vi "SVL AC & DC Level (1 Ch DBL WDT).vi"(9 "window":u16(ring)=8 items=["None ", "Hanning", "Hamming", "Blackman-Harris", "Exact Blackman", "Blackman", "Flat Top", "4 Term B-Harris ", "7 Term B-Harris", "Low Sidelobe"], 11 "scaled signal [EU]":waveform(dbl)={"t0"=timestamp(0 s since 1904-01-01), "dt"=0.0, "Y"=[]}) -> (1 "DC level [EU]":dbl=nan format="%0.2f", 2 "AC level [EU rms]":dbl=nan format="%.8f", 3 "AC signal [EU]":waveform(dbl))   [LabVIEW 2017]
doc: "Computes the AC level and DC level of a signal. Wire data to the <B>scaled signal [EU]</B> input to determine the polymorphic instance to use or manually select the instance."
uses:
  <vilib>/Analysis/baseanly.llb/Mean (DBL).vi
  <vilib>/Analysis/0measdsp.llb/Scaled Time Domain Window (DBL).vi
  <vilib>/Analysis/NI_AALBase.lvlib
  <vilib>/Analysis/NI_AALPro.lvlib
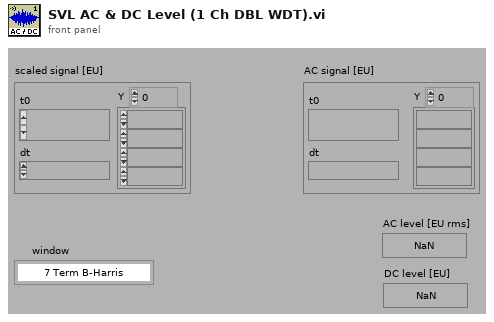
[diagram p1: front panel]
types:
  T1 = typedef "NI_AALPro.lvlib/windowTd.ctl" = u32
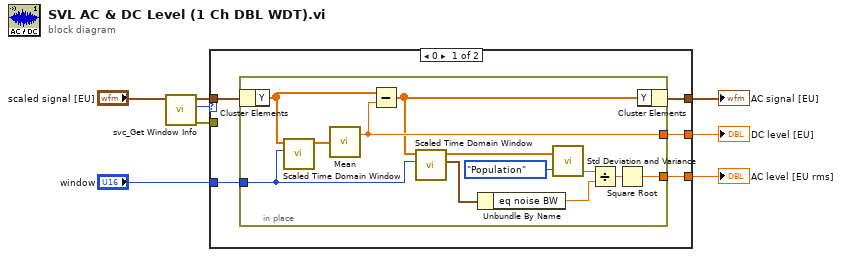
[diagram p0: block diagram]
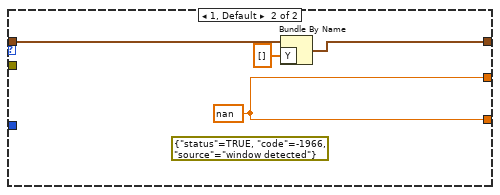
[diagram p2: hidden frame]
diagram:
  n1 = call <vilib>:"svc_Get Window Info.vi"("scaled signal [EU]"="scaled signal [EU]") -> ("error out"=w2:errorcluster, "window"=w1:T1, "dup scaled signal [EU]"=w3:waveform(dbl))  [unwired: 6 in, 2 out]
  n2 = case shown="0" w1 {
    tunnel: [w12 w29] -> w8
    tunnel: [w11 w29] -> w4
    tunnel: "window" -> [w13 _]
    tunnel: [w10 w27] -> w6
    tunnel: w3 -> [w9 w28]
    tunnel: w2 -> [_ _]
    frame 0 {
      n3 = in-place {
        in-place-border: [w19] -> w11
        in-place-border: w13 -> [w14]
        in-place-border: [w20] -> w12
        n4 = in-place-cluster #1(w9) -> ("Y"=w25:dbl[])
        n5 = call-poly <vilib>:"Scaled Time Domain Window.vi"("window"=w14, "X"=w25) -> ("Windowed X"=w18:dbl[])  [unwired: 7 in, 2 out]
        n6 = call-poly <vilib>:"Mean.vi"("X"=w18) -> ("mean"=w19:dbl)  [unwired: 1 out]
        n7 = Subtract(x=w25, y=w19) -> (x-y=w16:dbl[])
        n8 = call-poly <vilib>:"Scaled Time Domain Window.vi"("window"=w14, "X"=w16) -> ("window properties"=w15:cluster{"eq noise BW":dbl, "coherent gain":dbl}, "Windowed X"=w17:dbl[])  [unwired: 7 in, 1 out]
        n9 = Unbundle By Name(w15) -> ("eq noise BW"=w21:dbl)
        n10 = call <vilib>:"Std Deviation and Variance.vi"("X"=w17, "Weighting (Sample)"=enum16{"Sample", "Population"}."Population") -> ("variance"=w24:dbl)  [unwired: 2 out]
        n11 = Divide(x=w24, y=w21) -> (x/y=w22:dbl)
        n12 = Square Root(x=w22) -> (sqrt(x)=w20:dbl)
        n13 = in-place-cluster #1("Y"=w16) -> (w10:waveform(dbl))
      }
    }
    frame 1, Default {
      w29 = nan ("mean")
      (unwired) errorcluster {"status"=TRUE, "code"=-1966, "source"="window detected"} ("error in 2 (no error)")
      n14 = Bundle By Name(cluster=w28, "Y"=dbl[] []) -> (w27:waveform(dbl))
    }
  }
  "AC level [EU rms]" <- w8
  "DC level [EU]" <- w4
  "AC signal [EU]" <- w6
